vi "keithley reading-working.vi"() -> ()   [LabVIEW 2010]
panel:
  in  "stop":bool
  in  "VISA Resource Name":refnum<visa-resource-name>="GPIB0::2::INSTR"
  out "Read Buffer":string
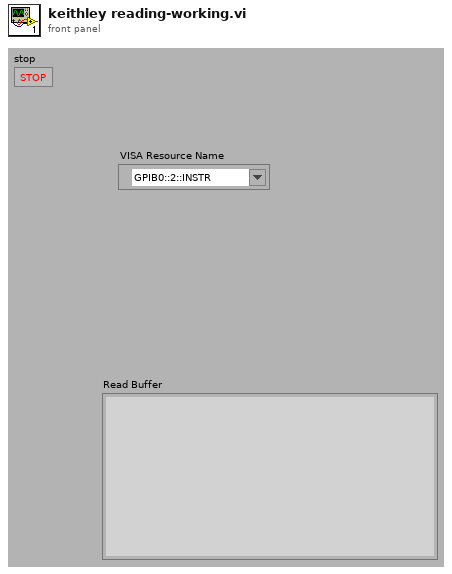
[diagram p1: front panel]
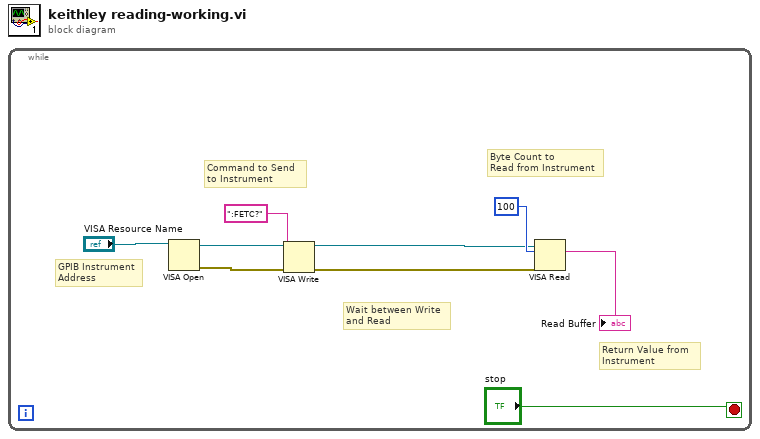
[diagram p0: block diagram]
diagram:
  n1 = while {
    stop <- "stop" stop-if-true
    # "Wait between Write\nand Read"
    # "Return Value from \nInstrument"
    # "Byte Count to\nRead from Instrument"
    # "Command to Send \nto Instrument"
    # "GPIB Instrument\nAddress"
    n2 = VISA Open(VISA resource name="VISA Resource Name") -> (VISA resource name=w1:refnum<visa-resource-name>, error out=w2:errorcluster)  [unwired: 4 in]
    n3 = VISA Write(VISA resource name=w1, write buffer=":FETC?" ("Write Buffer"), error in (no error)=w2) -> (VISA resource name out=w4:refnum<visa-resource-name>, error out=w3:errorcluster)  [unwired: 1 out]
    n4 = VISA Read(VISA resource name=w4, byte count=u32 100 ("Byte Count"), error in (no error)=w3) -> (read buffer=→"Read Buffer":string)  [unwired: 3 out]
  }
